vi "Host - ECAT Slaves write to XML-Log-File.vi"(6 "Operation (0:Öffnen)":T1(ring)=enum."replace or create", 7 "XML Log File name":string="VeriStand_ECAT_Logfile.xml", 8 "Fehler (Eingang, kein Fehler)":errorcluster, 11 "Referenz (Eingang)":refnum<k21>) -> (0 "Fehler (Ausgang)":errorcluster, 2 "Pfad":path, 3 "Referenz (Ausgang)":refnum<k21>)   [LabVIEW 2019, in "SEECD System Explorer.lvlib"]
uses:
  SEECD System Explorer.lvlib
  <vilib>/Utility/sysdir.llb/System Directory Type.ctl
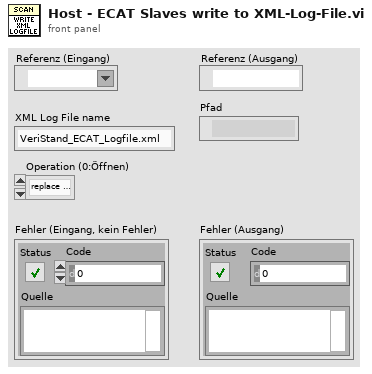
[diagram p1: front panel]
types:
  T1 = enum16{"open", "replace", "create", "open or create", "replace or create", "replace or create with confirmation"}
  T2 = typedef "System Directory Type.ctl" = i32
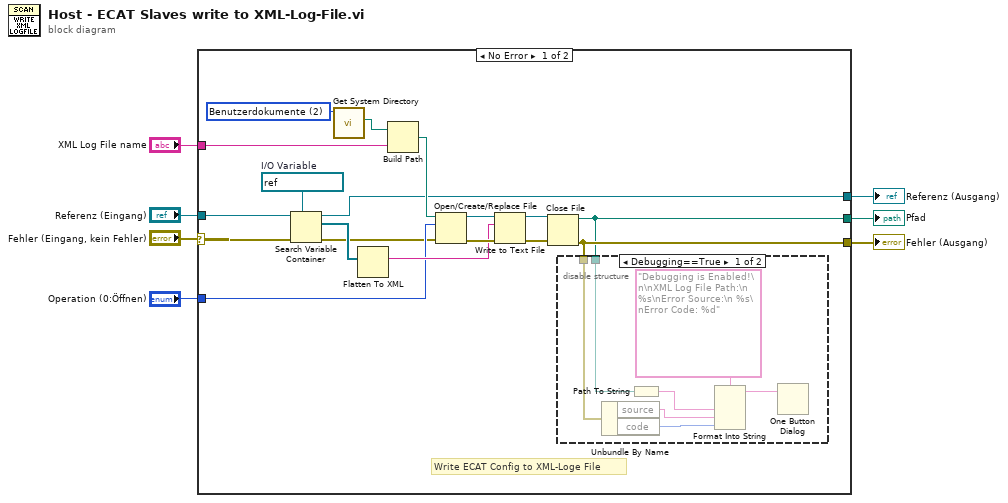
[diagram p0: block diagram]
diagram:
  n1 = case shown="No Error" "Fehler (Eingang, kein Fehler)" {
    selector: "Fehler (Eingang, kein Fehler)" -> [w13 w34]
    tunnel: [w12 w34] -> w7
    tunnel: "Operation (0:Öffnen)" -> [w20 _]
    tunnel: [w18 w33] -> w5
    tunnel: "Referenz (Eingang)" -> [w17 w33]
    tunnel: "XML Log File name" -> [w14 _]
    tunnel: [w11 _] -> w1
    frame No Error {
      w10 = T2 2 items=["Benutzerverzeichnis"=0, "Benutzer-Desktop"=1, "Benutzerdokumente"=2, "Benutzeranwendungsdaten"=3, "Benutzereinstellungen"=4, "Temporäres Verzeichnis"=5, "Öffentliche Dokumente"=6, "Öffentliche Anwendungsdaten"=7, "Öffentliche Einstellungen"=8, "Öffentlicher Cache"=13, "Systembibliotheken"=9, "Installierte Bibliotheken"=10, "Anwendungsdateien"=11, "Boot-Laufwerks-Stammverzeichnis"=12] ("system directory type")
      w16 = refnum<k21> refnum  # I/O Variable
      # "Write ECAT Config to XML-Loge File"
      n2 = Search Variable Container(7:w16, 8:w13, 11:w17) -> (0:w8:errorcluster, 2:w15:refnum<k21>[], 3:w18:refnum<k21>)  [unwired: 3 in]
      n3 = call <vilib>:"Get System Directory.vi"("system directory type"=w10) -> ("system directory"=w9:path)  [unwired: 10 in]
      n4 = Flatten To XML(anything=w15) -> (xml string=w22:string)
      n5 = Build Path(base path=w9, name or relative path=w14) -> (appended path=w19:path)
      n6 = Open/Create/Replace File(file path (use dialog)=w19, error in=w8, operation (0:open)=w20) -> (refnum out=w21:refnum<file>, error out=w23:errorcluster)  [unwired: 3 in, 1 out]
      n7 = Write to Text File(file (use dialog)=w21, text=w22, error in=w23) -> (refnum out=w25:refnum<file>, error out=w24:errorcluster)  [unwired: 1 in, 1 out]
      n8 = Close File(refnum=w25, error in=w24) -> (path=w11:path, error out=w12:errorcluster)
      n9 = disable-structure shown="Debugging==True" {
        disable-tunnel: w12 -> [w32 _]
        disable-tunnel: w11 -> [w31 _]
        frame condition #0 {
          n10 = Unbundle By Name(w32) -> ("source"=w28:string, "code"=w29:i32)
          n11 = Path To String(path=w31) -> (string=w27:string)
          n12 = Format Into String(format string="Debugging is Enabled!\n\nXML Log File Path:\n %s\nError Source:\n %s\nError Code: %d" ("Format-String"), w27, w28, w29) -> (resulting string=w26:string)  [unwired: 2 in, 1 out]
          n13 = One Button Dialog(message=w26) -> ()  [unwired: 1 in, 1 out]
        }
        frame condition #1 (active) {
        }
      }
    }
    frame Error {
    }
  }
  "Fehler (Ausgang)" <- w7
  "Referenz (Ausgang)" <- w5
  "Pfad" <- w1
